vi "PRL Data Reader.vi"(5 "Remove Bad Data?":bool, 7 "Queue Active?":bool, 9 "Initialize Data":T1, 10 "Initialize Time":bool, 11 "Initialize":bool) -> (0 "dt (ms)":dbl, 1 "Buffer Queued?":bool, 2 "Data Rate":dbl, 3 "Data?":bool, 4 "Bad Data?":bool, 6 "Bad Data Ratio":dbl, 8 "Latest Time Stamp":timestamp)   [LabVIEW 2018, in "S3DK.lvlib" / "PMU Recorder Light.lvlib"]
uses:
  PMU Recorder Light.lvlib
  Setting Choice.ctl
  Statnett C37.118 DLL/Statnett C37.118 DLL.lvclass
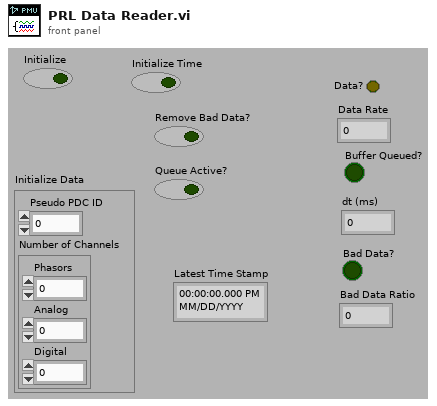
[diagram p1: front panel]
types:
  T1 = cluster{"Pseudo PDC ID":i32, "Number of Channels":cluster{"Phasors":i32, "Analog":i32, "Digital":i32}}
  T2 = cluster{"Phasors":i32, "Analog":i32, "Digital":i32}
  T3 = typedef "S3DK.lvlib/PMU Recorder Light.lvlib/Setting Choice.ctl" = enum16{"Analog Data Points Allowed Equals", "Complex Data Points Allowed Equals", "Seconds Before Reset After Wait for Config Fails", "Number of Live Buffer in Access Buffer ", "Number of Connection Attempts", "Live Data Buffer Size", "dt Tolerance", "Data Rate History", "ALL"}
  T4 = cluster{"dataErrorCode":u8, "pmuSyncFlag":u8, "pmuDataSortingFlag":u8, "pmuTriggerFlag":u8, "configChangeFlag":u8, "dataModifiedFlag":u8, "timeQualityCode":u8, "unlockTimeCode":u8, "triggerReasonCode":u8}[]
  T5 = cluster{"Time Stamp":timestamp, "Phasor Data":csg[], "Analog Data":sgl[], "Digital Data":bool[]}
  T6 = cluster{timestamp[], "Array Out":csg[][], "Array Out":sgl[][], bool[][], sgl[][]}
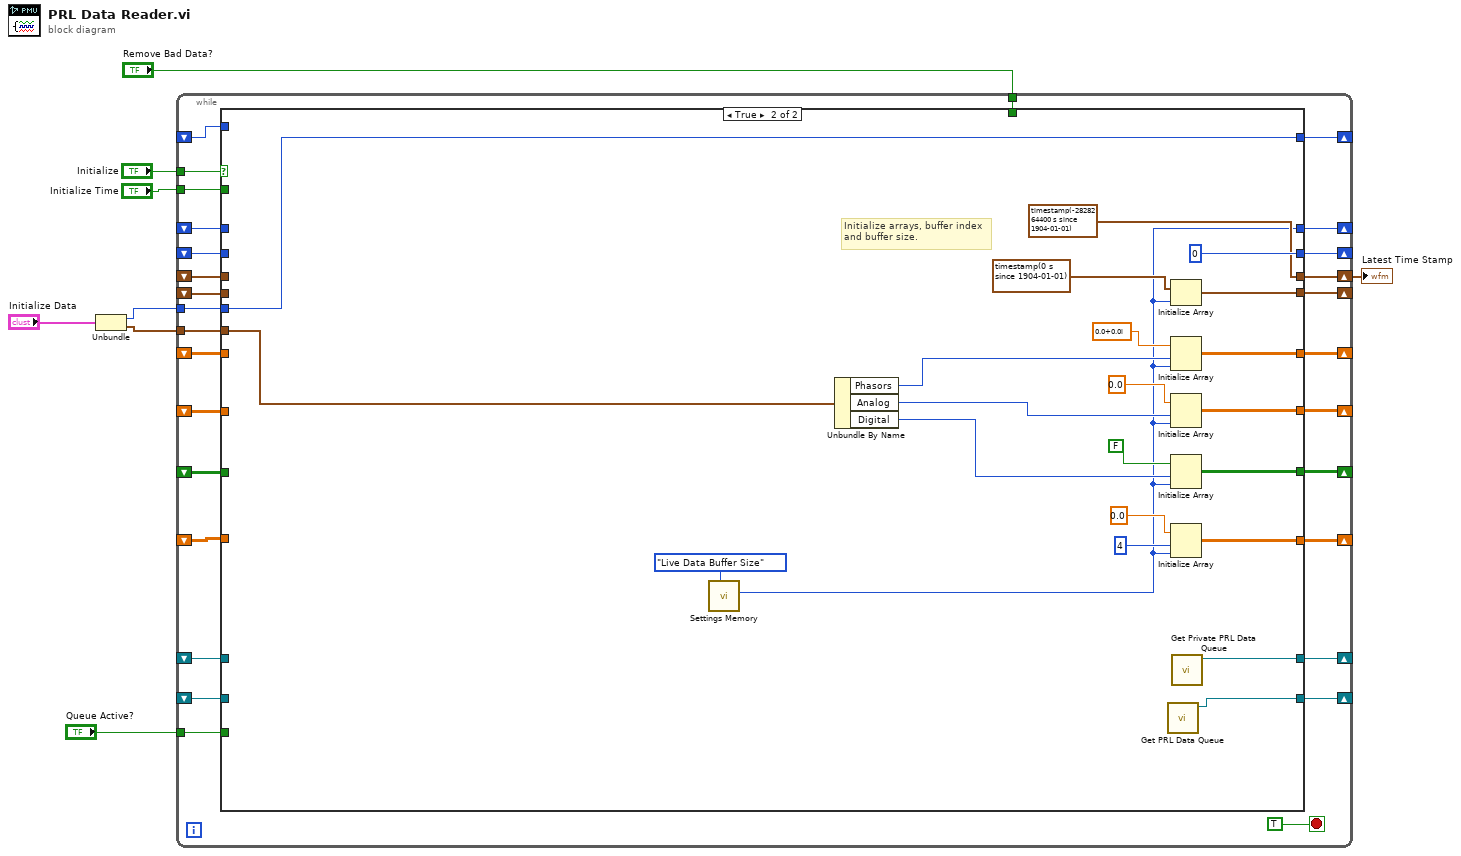
[diagram p0: block diagram]
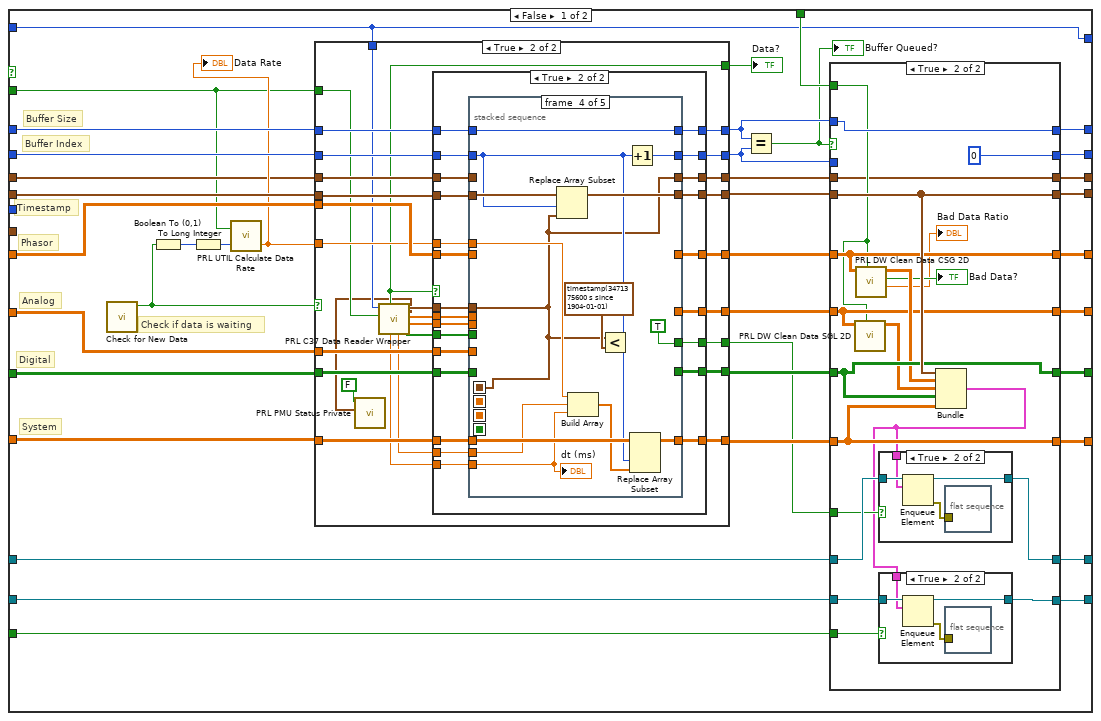
[diagram p2: hidden frame]
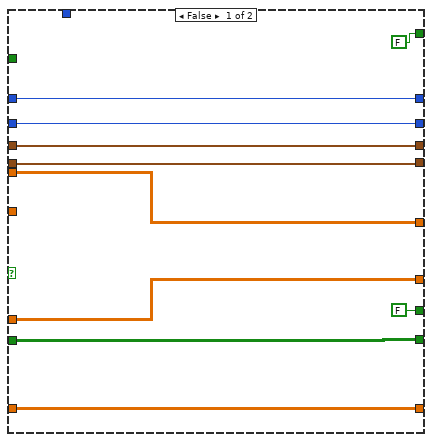
[diagram p3: hidden frame]
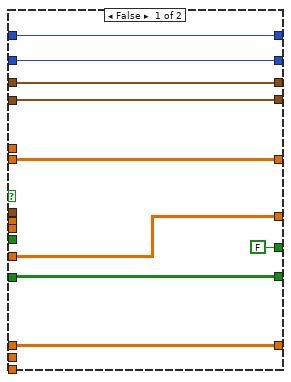
[diagram p4: hidden frame]
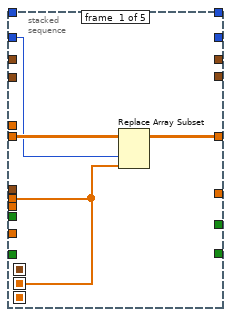
[diagram p5: hidden frame]
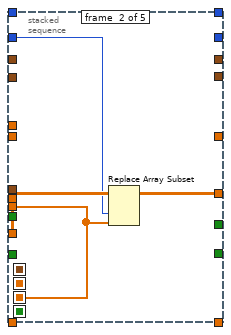
[diagram p6: hidden frame]
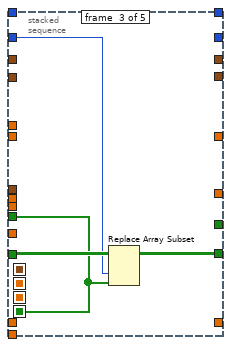
[diagram p7: hidden frame]
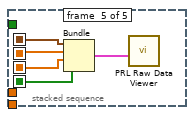
[diagram p8: hidden frame]
diagram:
  n1 = Unbundle("Initialize Data") -> ("Pseudo PDC ID"=w1:i32, "Number of Channels"=w2:T2)
  n2 = while {
    tunnel: w2 -> [w37]
    shift-right: [w25] -> _
    shift-left: _ -> [w35]
    shift-right: [w24] -> _
    shift-left: _ -> [w34]
    shift-right: [w23] -> _
    shift-left: _ -> [w33]
    shift-right: [w22] -> _
    shift-left: _ -> [w32]
    shift-right: [w21] -> _
    shift-left: _ -> [w31]
    tunnel: "Initialize" -> [w28]
    shift-right: [w26] -> _
    shift-left: _ -> [w30]
    shift-right: [w27] -> _
    shift-left: _ -> [w29]
    tunnel: "Initialize Time" -> [w18]
    shift-right: [w20] -> _
    shift-left: _ -> [w19]
    tunnel: "Remove Bad Data?" -> [w17]
    shift-right: [w16] -> _
    shift-left: _ -> [w15]
    tunnel: "Queue Active?" -> [w14]
    shift-right: [w12] -> w4
    shift-left: _ -> [w13]
    tunnel: w1 -> [w11]
    shift-right: [w10] -> _
    shift-left: _ -> [w9]
    stop <- TRUE stop-if-true
    n3 = case shown="True" w28 {
      tunnel: w37 -> [_ w227]
      tunnel: [w63 w233] -> w25
      tunnel: [w62 w232] -> w24
      tunnel: [w60 w231] -> w23
      tunnel: [w58 w230] -> w22
      tunnel: [w56 w229] -> w21
      tunnel: w35 -> [w74 _]
      tunnel: w34 -> [w73 _]
      tunnel: w33 -> [w72 _]
      tunnel: w32 -> [w71 _]
      tunnel: w31 -> [w70 _]
      tunnel: w30 -> [w75 _]
      tunnel: [w64 0 ("element")] -> w26
      tunnel: w29 -> [w76 _]
      tunnel: [w65 w220] -> w27
      tunnel: w18 -> [w42 _]
      tunnel: [w54 w226] -> w20
      tunnel: w19 -> [w55 _]
      tunnel: w17 -> [w53 _]
      tunnel: [w48 w224] -> w16
      tunnel: w15 -> [w49 _]
      tunnel: w14 -> [w47 _]
      tunnel: w13 -> [w46 _]
      tunnel: [w44 timestamp(-2828264400 s since 1904-01-01)] -> w12
      tunnel: w11 -> [_ w222]
      tunnel: [w41 w222] -> w10
      tunnel: w9 -> [w41 _]
      frame False {
        # "Check if data is waiting"
        # "System"
        # "Digital"
        # "Analog"
        # "Phasor"
        # "Timestamp"
        # "Buffer Index"
        # "Buffer Size"
        n4 = call "Check for New Data.vi"() -> ("Data Waiting"=w39:bool)  [unwired: 10 in, 1 out]
        n5 = Boolean To (0,1)(Boolean=w39) -> (0, 1=w43:i16)
        n6 = To Long Integer(number=w43) -> (32bit integer=w38:i32)
        n7 = call "PRL UTIL Calculate Data Rate.vi"("Data Indicator"=w38, "Init?"=w42) -> ("Data Rate"=w52:dbl)  [unwired: 1 out]
        "Data Rate" <- w52
        n8 = case shown="True" w39 {
          tunnel: w76 -> [w86 w115]
          tunnel: w75 -> [w85 w114]
          tunnel: w74 -> [w84 w113]
          tunnel: w73 -> [w83 w112]
          tunnel: w72 -> [w82 w111]
          tunnel: w71 -> [w81 w110]
          tunnel: w70 -> [w80 w109]
          tunnel: [w86 w108] -> w67
          tunnel: [w85 w107] -> w66
          tunnel: [w84 w106] -> w69
          tunnel: [w83 w105] -> w68
          tunnel: [w82 w104] -> w61
          tunnel: [w81 w103] -> w59
          tunnel: [w80 w101] -> w57
          tunnel: w52 -> [_ w102]
          tunnel: [FALSE w100] -> w50
          tunnel: w46 -> [w78 w99]
          tunnel: [w78 w98] -> w45
          tunnel: w42 -> [_ w91]
          tunnel: w41 -> [_ w90]
          tunnel: [FALSE ("Data OK") w89] -> w40
          frame False {
          }
          frame True {
            n9 = call "PRL C37 Data Reader Wrapper.vi"("Initialize Time"=w91, "Pseudo PDC ID"=w90) -> ("Digital Data"=w94:bool[], "Analog Data"=w95:sgl[], "Phasor Data"=w96:csg[], "Time Stamp"=w97:timestamp, "Relative System Clock (ms)"=w93:dbl, "PMU Status"=w88:T4, "dt (ms)"=w92:dbl, "Data OK"=w89:bool)  [unwired: 2 in]
            n10 = call "PRL PMU Status Private.vi"("PMU Status In"=w88, "Read(T)/Write(F)"=FALSE) -> ()  [unwired: 9 in, 1 out]
            n11 = case shown="True" w89 {
              tunnel: w115 -> [w116 w148]
              tunnel: w114 -> [w117 w147]
              tunnel: w113 -> [w119 w146]
              tunnel: w112 -> [w124 w145]
              tunnel: w111 -> [w123 w144]
              tunnel: w110 -> [w121 w143]
              tunnel: w109 -> [w120 w142]
              tunnel: [w116 w141] -> w108
              tunnel: [w117 w140] -> w107
              tunnel: [w119 w139] -> w106
              tunnel: [w124 w138] -> w105
              tunnel: [w123 w137] -> w104
              tunnel: [w121 w136] -> w103
              tunnel: w102 -> [_ w135]
              tunnel: [w120 w134] -> w101
              tunnel: [FALSE w133] -> w100
              tunnel: w99 -> [w118 w132]
              tunnel: [w118 w131] -> w98
              tunnel: w97 -> [_ w130]
              tunnel: w96 -> [_ w129]
              tunnel: w95 -> [_ w128]
              tunnel: w94 -> [_ w127]
              tunnel: w93 -> [_ w126]
              tunnel: w92 -> [_ w125]
              frame False {
              }
              frame True {
                n12 = stacked-sequence {
                  seq-local: [_ _ _ w162 _] -> [_ _ _ _ w179]
                  seq-local: [w149 _ _ _ _] -> [_ _ _ _ w178]
                  seq-local: [_ w153 _ _ _] -> [_ _ _ _ w177]
                  seq-local: [_ _ w157 _ _] -> [_ _ _ _ w176]
                  tunnel: w146 -> [_ _ _ w174 _]
                  tunnel: w145 -> [w152 _ _ _ _]
                  tunnel: w144 -> [_ w156 _ _ _]
                  tunnel: w143 -> [_ _ w160 _ _]
                  tunnel: w142 -> [_ _ _ w170 _]
                  tunnel: w147 -> [w151 w155 w158 w166 _]
                  tunnel: [w150 _ _ _ _] -> w138
                  tunnel: [_ w154 _ _ _] -> w137
                  tunnel: [_ _ w159 _ _] -> w136
                  tunnel: w148 -> [_ _ _ w172 _]
                  tunnel: [_ _ _ w173 _] -> w139
                  tunnel: [_ _ _ w172 _] -> w141
                  tunnel: [_ _ _ w171 _] -> w140
                  tunnel: w135 -> [_ _ _ w168 _]
                  tunnel: [_ _ _ w169 _] -> w134
                  tunnel: [_ _ _ TRUE _] -> w133
                  tunnel: w132 -> [_ _ _ _ _]
                  tunnel: [_ _ _ w162 _] -> w131
                  tunnel: w129 -> [w149 _ _ _ _]
                  tunnel: w128 -> [_ w153 _ _ _]
                  tunnel: w127 -> [_ _ w157 _ _]
                  tunnel: w126 -> [_ _ _ w164 _]
                  tunnel: w125 -> [_ _ _ w163 _]
                  tunnel: w130 -> [_ _ _ w162 _]
                  frame #0 {
                    n13 = Replace Array Subset(array=w152, new element=w149, index (col)=w151) -> (w150:csg[][])  [unwired: 1 in]
                  }
                  frame #1 {
                    n14 = Replace Array Subset(array=w156, new element=w153, index (col)=w155) -> (w154:sgl[][])  [unwired: 1 in]
                  }
                  frame #2 {
                    n15 = Replace Array Subset(array=w160, new element=w157, index (col)=w158) -> (w159:bool[][])  [unwired: 1 in]
                  }
                  frame #3 {
                    n16 = Replace Array Subset(array=w174, new element=w162, index=w166) -> (w173:timestamp[])
                    n17 = Build Array(w168, w164, w163) -> (w167:dbl[])
                    n18 = Less?(x=w162, y=timestamp(3471375600 s since 1904-01-01)) -> ()  [unwired: 1 out]
                    n19 = Increment(x=w166) -> (x+1=w171:i32)
                    n20 = Replace Array Subset(array=w170, new element=w167, index (col)=w166) -> (w169:sgl[][])  [unwired: 1 in]
                    "dt (ms)" <- w163
                  }
                  frame #4 {
                    n21 = Bundle("Time Stamp"=w179, "Phasor Data"=w178, "Analog Data"=w177, "Digital Data"=w176) -> (w175:T5)  [unwired: 1 in]
                    n22 = call "PRL Raw Data Viewer.vi"("Raw Data"=w175) -> ()  [unwired: 11 in]
                  }
                }
              }
            }
          }
        }
        "Data?" <- w40
        n23 = Equal?(x=w67, y=w66) -> (x = y?=w51:bool)
        "Buffer Queued?" <- w51
        n24 = case shown="True" w51 {
          tunnel: w67 -> [w189 w209]
          tunnel: w66 -> [w188 _]
          tunnel: w69 -> [w187 w205]
          tunnel: w68 -> [w186 w202]
          tunnel: [w189 w209] -> w65
          tunnel: [w188 0 ("Data Buffer Size")] -> w64
          tunnel: [w187 w205] -> w63
          tunnel: [w186 w202] -> w62
          tunnel: w61 -> [w185 w198]
          tunnel: [w185 w198] -> w60
          tunnel: w59 -> [w184 w204]
          tunnel: [w184 w204] -> w58
          tunnel: w57 -> [w183 w203]
          tunnel: [w183 w203] -> w56
          tunnel: w55 -> [w182 w207]
          tunnel: [w182 w206] -> w54
          tunnel: w53 -> [_ w196]
          tunnel: w50 -> [_ w195]
          tunnel: w49 -> [w181 w194]
          tunnel: [w181 w193] -> w48
          tunnel: w47 -> [_ w191]
          tunnel: w45 -> [w180 w190]
          tunnel: [w180 w190] -> w44
          frame False {
          }
          frame True {
            n25 = call "PRL DW Clean Data SGL 2D.vi"("Remove Bad Data?"=w196, "Array In"=w198) -> ("Array Out"=w197:sgl[][])  [unwired: 7 in, 2 out]
            n26 = call "PRL DW Clean Data CSG 2D.vi"("Remove Bad Data?"=w196, "Array In"=w202) -> ("Bad Data Ratio"=→"Bad Data Ratio":dbl, "Bad Data?"=→"Bad Data?":bool, "Array Out"=w201:csg[][])  [unwired: 7 in]
            n27 = Bundle(w205, "Array Out"=w201, "Array Out"=w197, w204, w203) -> (w192:T6)  [unwired: 1 in]
            n28 = case shown="True" w195 {
              tunnel: w207 -> [w215 w219]
              tunnel: w192 -> [_ w218]
              tunnel: [w215 w217] -> w206
              frame False {
              }
              frame True {
                n29 = Enqueue Element(queue=w219, element=w218) -> (queue out=w217:refnum<queue>, error out=w216:errorcluster)  [unwired: 2 in, 1 out]
                n30 = flat-sequence {
                  tunnel: w216 -> [_]
                  frame #0 {
                  }
                }
              }
            }
            n31 = case shown="True" w191 {
              tunnel: w194 -> [w210 w214]
              tunnel: w192 -> [_ w213]
              tunnel: [w210 w212] -> w193
              frame False {
              }
              frame True {
                n32 = Enqueue Element(queue=w214, element=w213) -> (queue out=w212:refnum<queue>, error out=w211:errorcluster)  [unwired: 2 in, 1 out]
                n33 = flat-sequence {
                  tunnel: w211 -> [_]
                  frame #0 {
                  }
                }
              }
            }
          }
        }
      }
      frame True {
        # "Initialize arrays, buffer index\nand buffer size."
        n34 = call "Settings Memory.vi"("Setting Choice"=Setting_Choice."Live Data Buffer Size") -> ("Output Int32"=w220:i32)  [unwired: 8 in, 2 out]
        n35 = Unbundle By Name(w227) -> ("Phasors"=w236:i32, "Analog"=w235:i32, "Digital"=w234:i32)
        n36 = call "Get PRL Data Queue.vi"() -> ("PRL Data Queue"=w224:refnum<queue>)  [unwired: 11 in]
        n37 = Initialize Array(timestamp(0 s since 1904-01-01), w220) -> (w233:timestamp[])
        n38 = Initialize Array(csg 0.0+0.0i ("element"), w236, w220) -> (w232:csg[][])
        n39 = Initialize Array(sgl 0.0 ("element"), w235, w220) -> (w231:sgl[][])
        n40 = Initialize Array(FALSE, w234, w220) -> (w230:bool[][])
        n41 = Initialize Array(sgl 0.0 ("element"), 4 ("dimension size"), w220) -> (w229:sgl[][])
        n42 = call "Get Private PRL Data Queue.vi"() -> ("PRL Data Queue"=w226:refnum<queue>)  [unwired: 11 in]
      }
    }
  }
  "Latest Time Stamp" <- w4
